vi "Measure, Analyze, and Save I-V of Diodes.vi"() -> ()   [LabVIEW 2020]
doc: "Measure, Analyze, and Save I-V of Diodes.vi contains a state machine that is meant to measure, analyze, and save the I-V characteristics of a diode in series with a resistor on a breadboard using the NI myDAQ data acquisition device. The channel AO0 is used to output a voltage to the breadboard, AI0 is used the measure the voltage across the resistor, and AI1 is used to measure the voltage across the diode. The states are as follows:\n\nInitialize Specifications for Measurement: \nThe user is prompted if they want to input their own measurement specifications or demo the VI with recommended values (for either the linear or log case). The inputted values are checked so that the diode is not put in danger. If the inputted values are safe, the user is sent to the Pre-Measurement state. Otherwise, they are sent to the Input Error state.\n\nPre-Measurement (Calculate Voltage Array):\nThe input values are used to create an array of voltages using the \"Calculate Voltage Array\" sub VI that will be sent to the output of the NI myDAQ device. If the voltage is high enough to exceed the peak current, the creation of the array will cease. Then the user is sent to the Measurement state.\n\nMeasurement:\nThe inputted values are sent the the \"Measure I-V of Diodes\" sub VI. The output voltage, current, and diode voltage measurements are outputted as an array indicator and are plotted to the XY Graph \"I (mA) vs. V_Diode (V)\". A value of 0 V is then dent to the NI myDAQ to turn off the LED after all measurements have been collected. The data is sent to the \"Format Data String\" sub VI which formats the data into a comma-separated values file. The user is prompted on whether they want to choose the filename and path for the saved data or have a default name and path chosen for them. The file path is outputted as an indicator and the user is prompted to either go to the Analysis state or Reset Values and Restart/Stop state.\n\nAnalysis:\nThe current measurements are sent to the \"Indices of Negative Array Elements\" sub VI. The outputted array containing the indices of the negative current values and the voltages are both sent to the \"Remove Elements from Array by Index\" sub VI, which removes any data points with negative current so that they are not out of range for the logarithm of base 10 function. The logarithm of base 10 of the current is then calculated and plotted against the voltage values in the \"Log ( I ( mA ) ) vs. V_Diode ( V )\" XY Graph. A linear best fit is also calculated and plotted. The slope and y-intercept from the best fit line are used to calculate the ideality factor and forward voltage when the current is 1.5 mA. The user is then sent to the Reset Values and Restart/Stop state.\n\nReset Values and Restart/Stop:\nThe user is prompted if they want to restart or stop the state machine. All front panel indicator values are reset.\n\nInput Error:\nThe user is notified that there was an error with their input. Then the state machine restarts."
uses:
  VI State Enum Type Def.ctl
  <vilib>/DAQmx/write.llb/DAQmx Write (Analog DBL 1Chan 1Samp).vi
  <vilib>/DAQmx/create/channels.llb/DAQmx Create Channel (AO-Voltage-Basic).vi
  <vilib>/DAQmx/create/channels.llb/DAQmx Create Channel (AI-Voltage-Basic).vi
  <vilib>/DAQmx/miscellaneous.llb/DAQmx Fill In Error Info.vi
  <vilib>/Analysis/NI_AALPro.lvlib
panel:
  out "Filename Out":path
  out "Room Temperature (K)":dbl
  out "Boltzmann Constant (J/K)":dbl
  out "Electron Charge (C)":dbl
  out "Saturation Current (mA)":dbl
  out "Ideality Factor":dbl
  out "V_F @ 1.5 mA (V)":dbl
  out "Coefficient of Determination":dbl
  out "Y-Intercept":dbl
  out "Slope":dbl
  out "Log ( I (mA) ) vs. V_Diode (V)":cluster{"Y":dbl[], "Y":dbl[]}[](graph)
  out "I (mA) vs. V_Diode (V)":cluster{"Y":dbl[], "Y":dbl[]}[](graph)
  out "I/O Array":dbl[][](array[numeric])
  in  "Stop Measurement":bool
  out "Measurement Specifications":T1
  in  "Stop VI":bool
  # "Measure I-V of Diodes"
  # "V_Applied (V)"
  # "I (mA)"
  # "V_Diode (V)"
  # "Analyze I-V of Diodes"
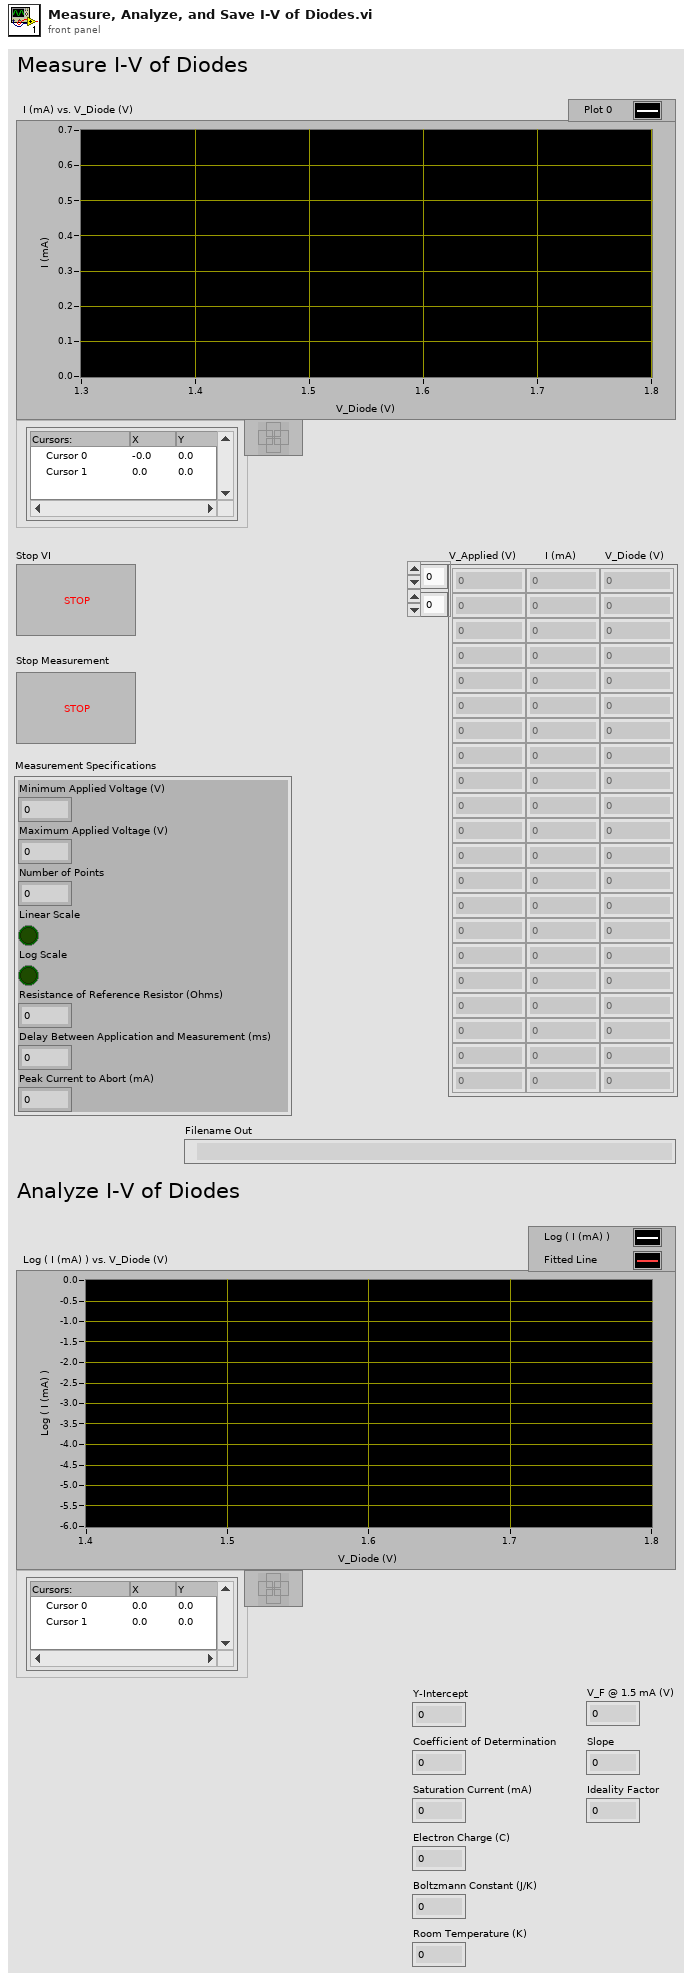
[diagram p1: front panel]
types:
  T1 = cluster{"Minimum Applied Voltage (V)":dbl, "Maximum Applied Voltage (V)":dbl, "Number of Points":i32, "Linear Scale":bool, "Log Scale":bool, "Resistance of Reference Resistor (Ohms)":dbl, "Delay Between Application and Measurement (ms)":dbl, "Peak Current to Abort (mA)":dbl}
  T2 = cluster{"Minimum Applied Voltage (V) (-10 V <= V_min <= 0 V)":dbl, "Maximum Applied Voltage (V) (0 V < V_max <= 10 V)":dbl, "Number of Points to Measure (Integer)":dbl, "Linear Scale":bool, "Log Scale":bool, "Resistance of the Reference Resistor (Ohms)":dbl, "Delay Between Application and Measurement (ms)":dbl, "Peak Current to Abort (mA)":dbl}
  T3 = typedef "VI State Enum Type Def.ctl" = enum16{"Initialize Specifications for Measurement", "Pre-Measurement (Calculate Voltage Array)", "Measurement", "Analysis", "Reset Values and Restart/Stop", "Input Error"}
  T4 = enum16{"open", "replace", "create", "open or create", "replace or create", "replace or create with confirmation"}
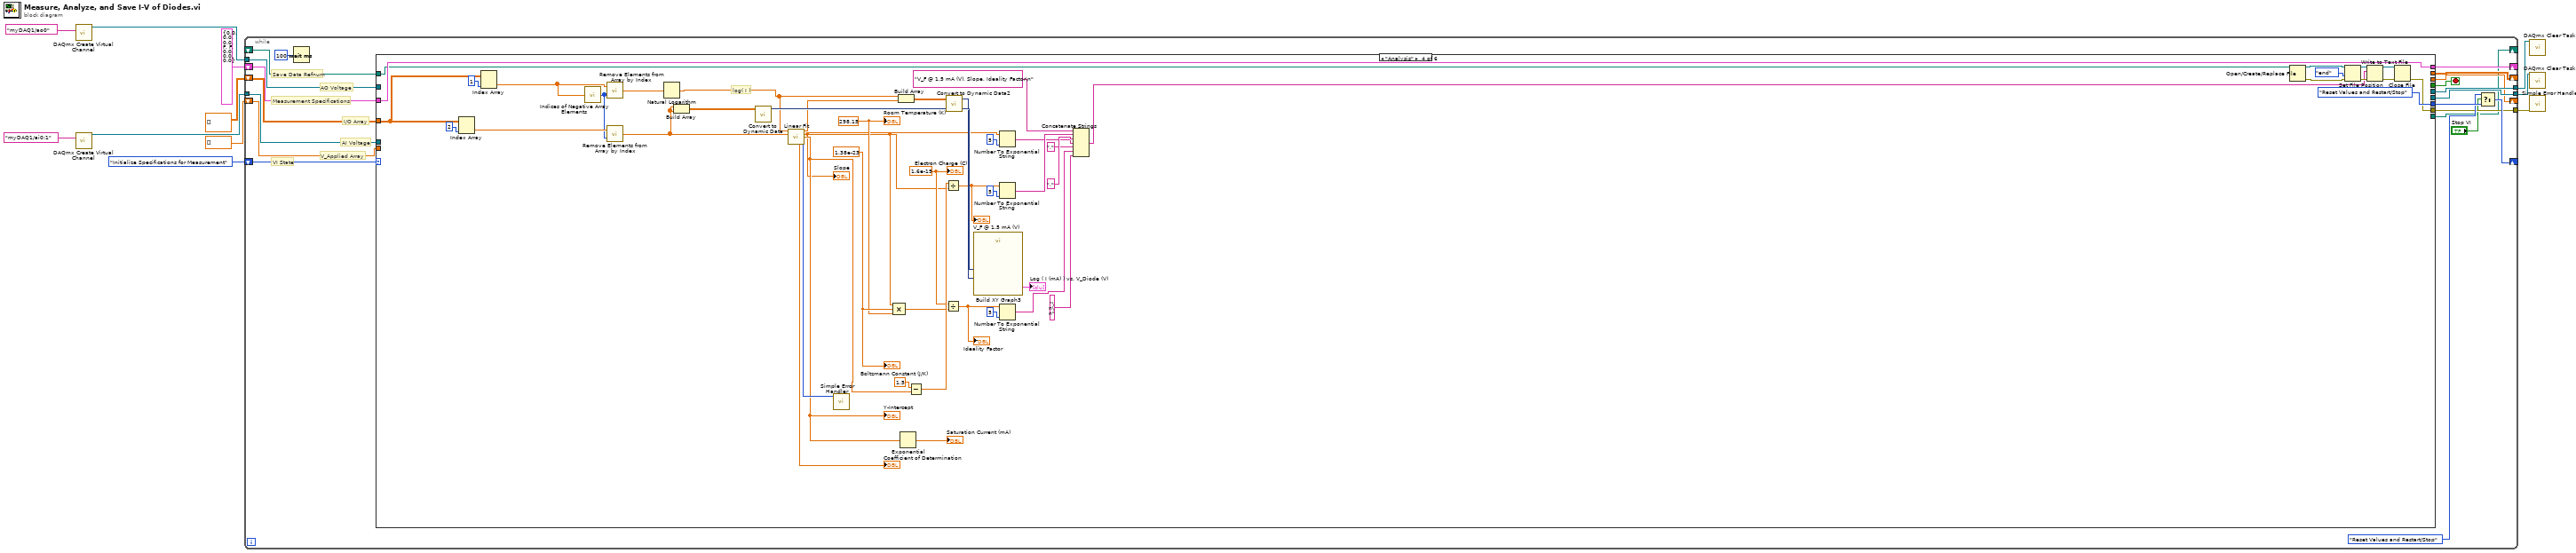
[diagram p0: block diagram]
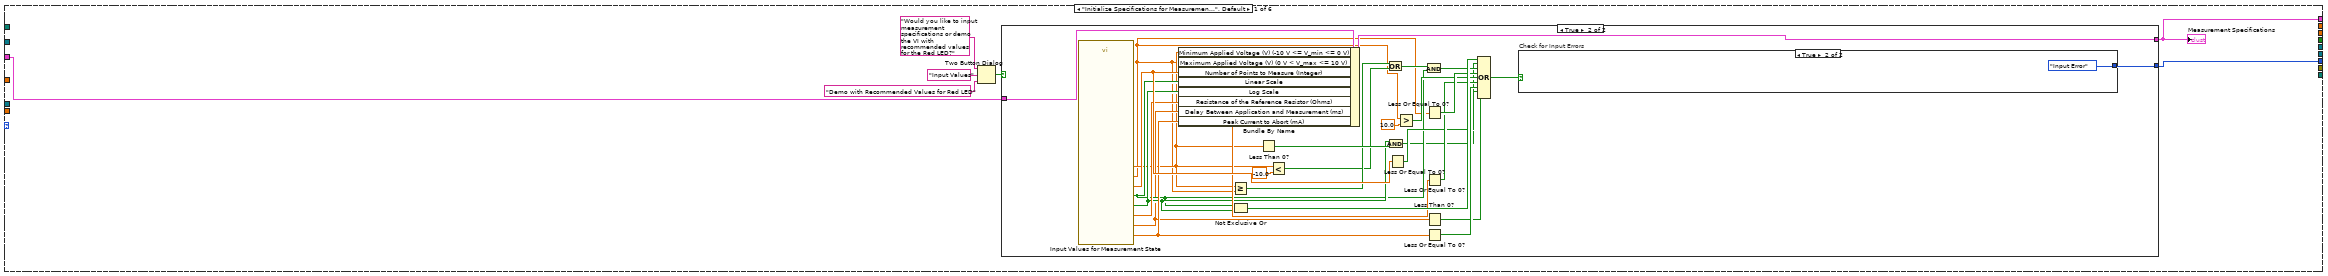
[diagram p2: hidden frame]
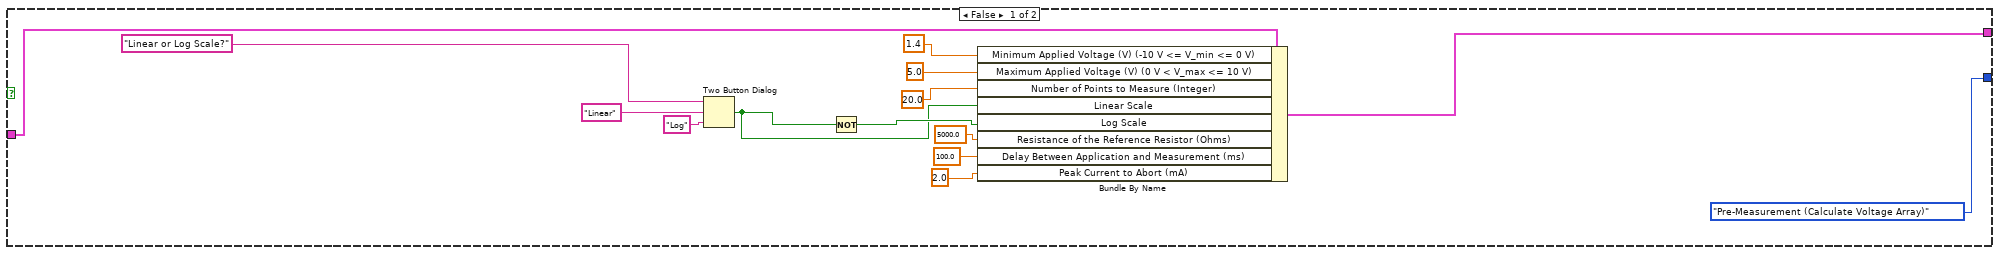
[diagram p3: hidden frame]
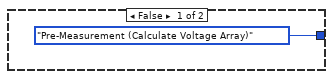
[diagram p4: hidden frame]
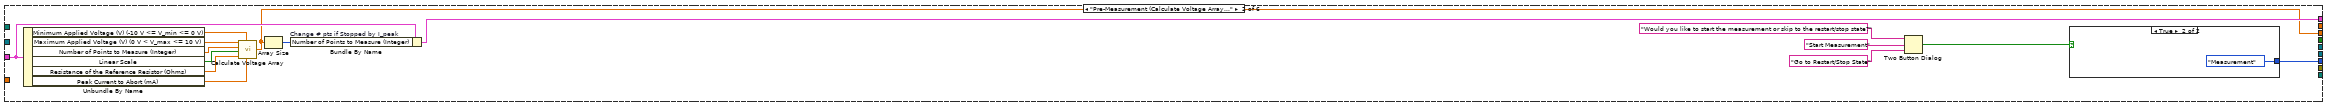
[diagram p5: hidden frame]
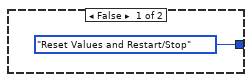
[diagram p6: hidden frame]
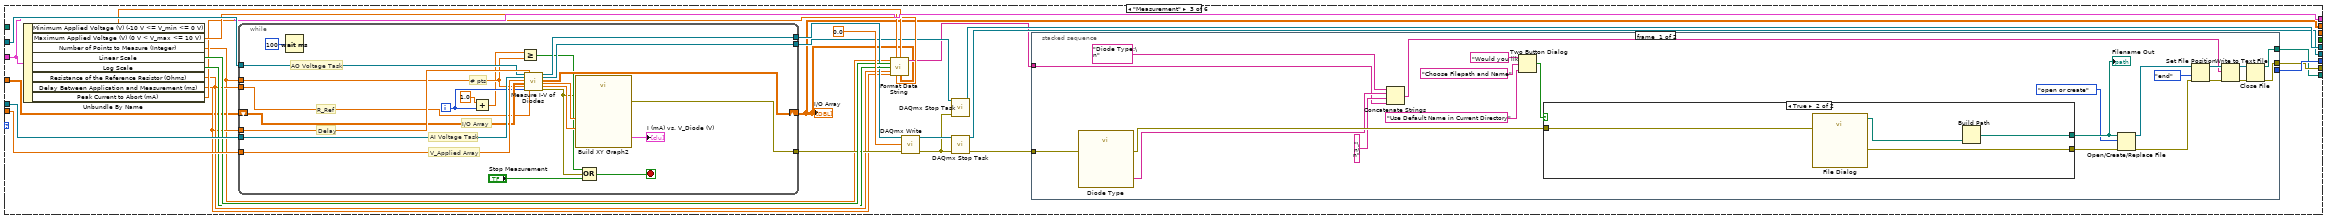
[diagram p7: hidden frame]
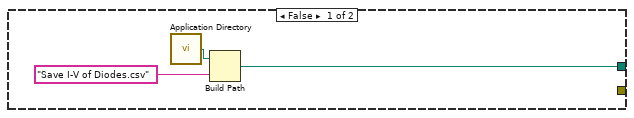
[diagram p8: hidden frame]
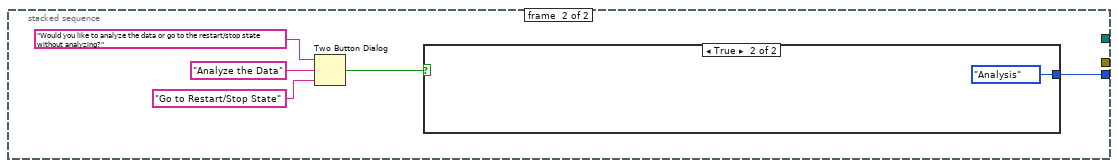
[diagram p9: hidden frame]
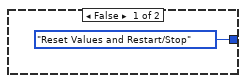
[diagram p10: hidden frame]
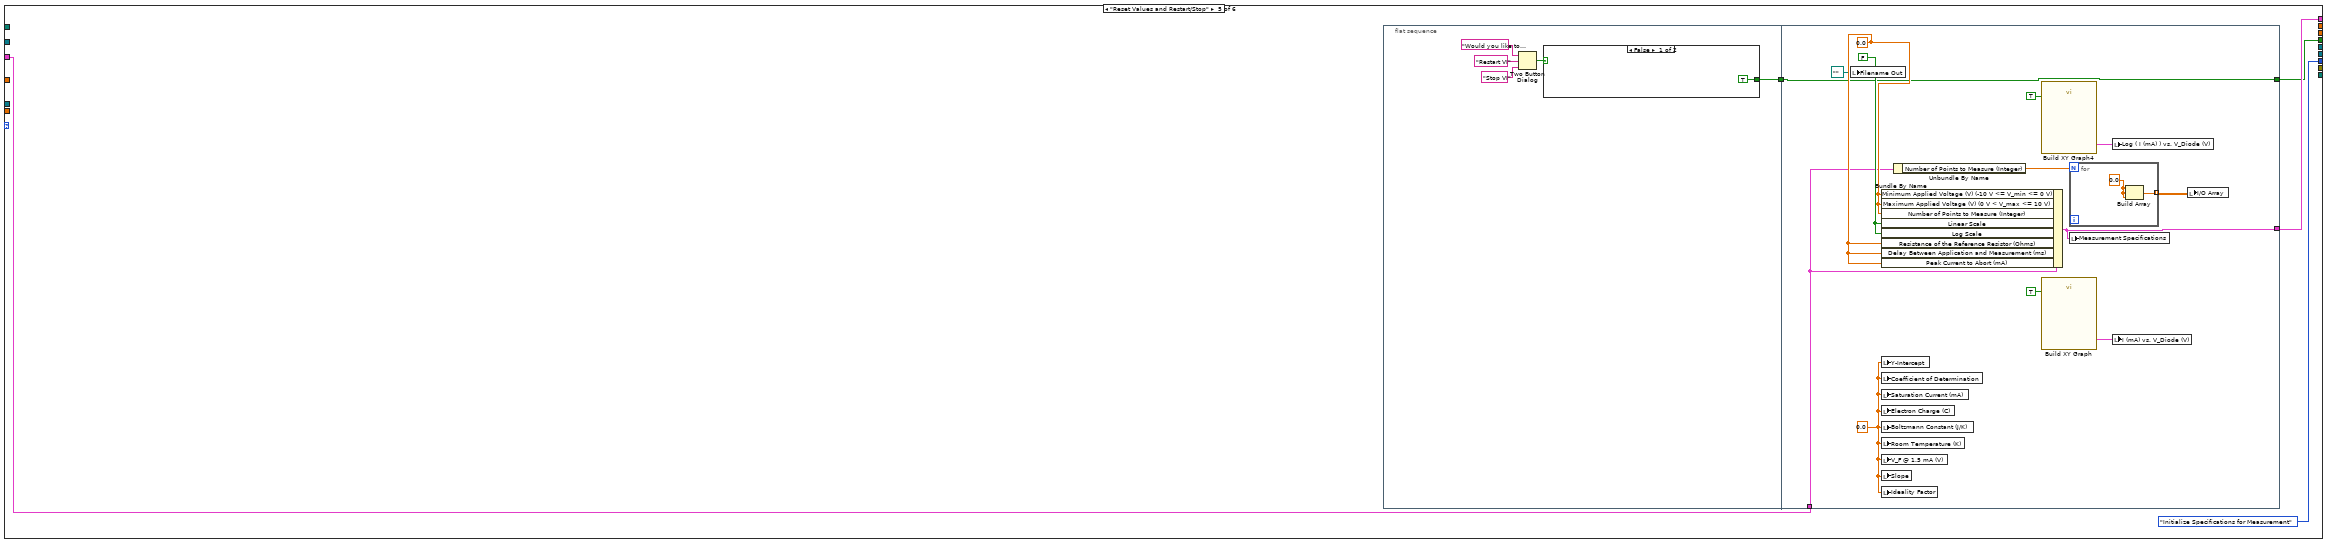
[diagram p11: hidden frame]
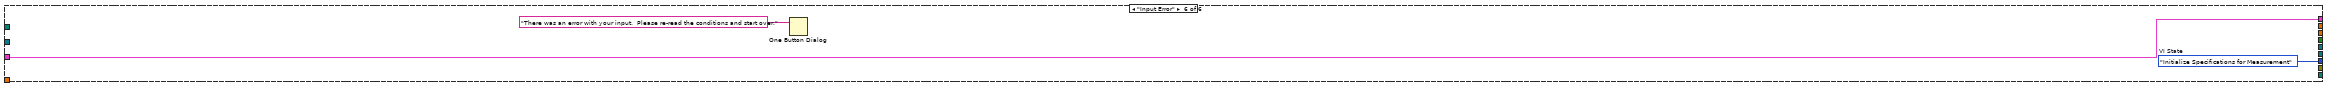
[diagram p13: hidden frame]
diagram:
  n1 = call-poly <vilib>:"DAQmx Create Virtual Channel.vi"("physical channels"=tag "myDAQ1/ao0") -> ("task out"=w5:refnum<k21>)  [unwired: 13 in, 1 out]
  n2 = call-poly <vilib>:"DAQmx Create Virtual Channel.vi"("physical channels"=tag "myDAQ1/ai0:1") -> ("task out"=w8:refnum<k21>)  [unwired: 13 in, 1 out]
  n3 = while {
    shift-right: [w22] -> _
    shift-left: VI_State_Enum_Type_Def."Initialize Specifications for Measurement" ("VI State") -> [w31]
    tunnel: w5 -> [w29]
    tunnel: w8 -> [w28]
    tunnel: [w27] -> w7
    tunnel: [w26] -> w6
    shift-right: [w25] -> _
    shift-left: T2 {"Minimum Applied Voltage (V) (-10 V <= V_min <= 0 V)"=0.0, "Maximum Applied Voltage (V) (0 V < V_max <= 10 V)"=0.0, "Number of Points to Measure (Integer)"=0.0, "Linear Scale"=FALSE, "Log Scale"=FALSE, "Resistance of the Reference Resistor (Ohms)"=0.0, "Delay Between Application and Measurement (ms)"=0.0, "Peak Current to Abort (mA)"=0.0} -> [w24]
    shift-right: [w20] -> _
    shift-left: dbl[] [] ("Voltage Array") -> [w19]
    tunnel: [w18] -> w2
    shift-right: [w17] -> _
    shift-left: dbl[][] [] ("I/O Array Out") -> [w16]
    shift-right: [w13] -> _
    shift-left: _ -> [w12]
    stop <- w15 stop-if-true
    # "Save Data Refnum"
    # "I/O Array"
    # "V_Applied Array"
    # "Measurement Specifications"
    # "AI Voltage"
    # "AO Voltage"
    # "VI State"
    n4 = Wait (ms)(milliseconds to wait=u32 100) -> ()  [unwired: 1 out]
    n5 = case shown="\"Analysis\"" w31 {
      tunnel: [w38 w96 w108 VI_State_Enum_Type_Def."Reset Values and Restart/Stop" ("Measurement State") VI_State_Enum_Type_Def."Initialize Specifications for Measurement" ("VI State") w262] -> w23
      tunnel: w29 -> [_ _ w123 _ _ _]
      tunnel: w28 -> [_ _ w122 _ _ _]
      tunnel: [_ _ w125 _ _ _] -> w27
      tunnel: [_ _ w124 _ _ _] -> w26
      tunnel: [w36 w93 w118 w233 w239 w261] -> w25
      tunnel: w24 -> [w37 w95 w118 w233 w238 w261]
      tunnel: [_ w86 _ _ _ _] -> w20
      tunnel: w19 -> [_ _ w119 _ _ _]
      tunnel: [_ _ w106 w185 _ _] -> w18
      tunnel: [_ _ w101 _ _ _] -> w17
      tunnel: w16 -> [_ _ w100 w231 _ _]
      tunnel: [_ _ _ _ w235 _] -> w15
      tunnel: [_ _ w99 _ _ _] -> w13
      tunnel: w12 -> [_ _ _ w207 _ _]
      frame "Initialize Specifications for Measurement", Default {
        n6 = Two Button Dialog(message="Would you like to input measurement specifications or demo the VI with recommended values for the Red LED?", 1:"Demo with Recommended Values for Red LED" ("F button name (\"Cancel\")"), 2:"Input Values" ("T button name (\"OK\")")) -> (T button?=w32:bool)
        n7 = case shown="True" w32 {
          tunnel: [VI_State_Enum_Type_Def."Pre-Measurement (Calculate Voltage Array)" ("VI State") w79] -> w38
          tunnel: w37 -> [w52 w70]
          tunnel: [w46 w66] -> w36
          frame False {
            n8 = Two Button Dialog(message="Linear or Log Scale?", 1:"Log" ("F button name (\"Cancel\")"), 2:"Linear" ("T button name (\"OK\")")) -> (T button?=w40:bool)
            n9 = Not(x=w40) -> (.not. x?=w41:bool)
            n10 = Bundle By Name(cluster=w52, "Minimum Applied Voltage (V) (-10 V <= V_min <= 0 V)"=1.4, "Maximum Applied Voltage (V) (0 V < V_max <= 10 V)"=5.0, "Number of Points to Measure (Integer)"=20.0, "Linear Scale"=w40, "Log Scale"=w41, "Resistance of the Reference Resistor (Ohms)"=5000.0, "Delay Between Application and Measurement (ms)"=100.0, "Peak Current to Abort (mA)"=2.0) -> (w46:T2)
          }
          frame True {
            n11 = call "Input Values for Measurement State"() -> ("Peak Current to Abort (mA) (I_peak > 0 mA)"=w67:dbl, "Delay Between Application and Measurement (ms) (Delay >= 0 ms)"=w56:dbl, "Resistance of the Reference Resistor (Ohms) (R_ref > 0 Ohms)"=w68:dbl, "Log Scale"=w64:bool, "Linear Scale"=w59:bool, "Number of Points to Measure (Integer) (# pts > 0)"=w69:dbl, "Maximum Applied Voltage (V) (0 V < V_max <= 10 V)"=w53:dbl, "Minimum Applied Voltage (V) (See Above for Conditions)"=w54:dbl)  [unwired: 10 in, 2 out]
            n12 = Bundle By Name(cluster=w70, "Minimum Applied Voltage (V) (-10 V <= V_min <= 0 V)"=w54, "Maximum Applied Voltage (V) (0 V < V_max <= 10 V)"=w53, "Number of Points to Measure (Integer)"=w69, "Linear Scale"=w59, "Log Scale"=w64, "Resistance of the Reference Resistor (Ohms)"=w68, "Delay Between Application and Measurement (ms)"=w56, "Peak Current to Abort (mA)"=w67) -> (w66:T2)
            n13 = Greater Or Equal?(x=w54, y=w53) -> (x >= y?=w63:bool)
            n14 = Not Exclusive Or(1:w64, 2:w59) -> (0:w78:bool)
            n15 = Less Than 0?(x=w54) -> (x < 0?=w65:bool)
            n16 = Less?(x=w54, y=-10.0) -> (x < y?=w62:bool)
            n17 = Or(x=w63, y=w62) -> (x .or. y?=w60:bool)
            n18 = And(x=w64, y=w65) -> (x .and. y?=w55:bool)
            n19 = Less Or Equal To 0?(x=w69) -> (x <= 0?=w71:bool)
            n20 = Greater?(x=w53, y=10.0) -> (0:w74:bool)
            n21 = And(x=w60, y=w59) -> (x .and. y?=w58:bool)
            n22 = Less Or Equal To 0?(x=w53) -> (x <= 0?=w76:bool)
            n23 = Less Or Equal To 0?(x=w68) -> (x <= 0?=w73:bool)
            n24 = Less Than 0?(x=w56) -> (x < 0?=w57:bool)
            n25 = Less Or Equal To 0?(x=w67) -> (x <= 0?=w72:bool)
            n26 = Compound Arithmetic op=OR(w78, w55, w58, w76, w74, w73, w72, w71, w57) -> (w77:bool)
            n27 = case "Check for Input Errors" shown="True" w77 {
              tunnel: [VI_State_Enum_Type_Def."Pre-Measurement (Calculate Voltage Array)" ("Measurement State") VI_State_Enum_Type_Def."Input Error" ("Measurement State")] -> w79
              frame False {
              }
              frame True {
              }
            }
          }
        }
        "Measurement Specifications" <- w36
      }
      frame "Pre-Measurement (Calculate Voltage Array)" {
        n28 = Unbundle By Name(w95) -> ("Minimum Applied Voltage (V) (-10 V <= V_min <= 0 V)"=w92:dbl, "Maximum Applied Voltage (V) (0 V < V_max <= 10 V)"=w91:dbl, "Number of Points to Measure (Integer)"=w90:dbl, "Linear Scale"=w89:bool, "Resistance of the Reference Resistor (Ohms)"=w88:dbl, "Peak Current to Abort (mA)"=w87:dbl)
        n29 = call "Calculate Voltage Array.vi"("I_peak"=w87, "V_min"=w92, "R_ref"=w88, "Scale (True == Linear, False == Log)"=w89, "# pts"=w90, "V_max"=w91) -> ("Voltage Array"=w86:dbl[])
        n30 = Array Size(array=w86) -> (size(s)=w94:i32)
        n31 = Bundle By Name "Change # pts if Stopped by I_peak"(cluster=w95, "Number of Points to Measure (Integer)"=w94) -> (w93:T2)
        n32 = Two Button Dialog(message="Would you like to start the measurement or skip to the restart/stop state?", 1:"Go to Restart/Stop State" ("F button name (\"Cancel\")"), 2:"Start Measurement" ("T button name (\"OK\")")) -> (T button?=w85:bool)
        n33 = case shown="True" w85 {
          tunnel: [VI_State_Enum_Type_Def."Reset Values and Restart/Stop" ("Measurement State") VI_State_Enum_Type_Def."Measurement" ("Measurement State")] -> w96
          frame False {
          }
          frame True {
          }
        }
      }
      frame "Measurement" {
        n34 = Unbundle By Name(w118) -> ("Minimum Applied Voltage (V) (-10 V <= V_min <= 0 V)"=w117:dbl, "Maximum Applied Voltage (V) (0 V < V_max <= 10 V)"=w116:dbl, "Number of Points to Measure (Integer)"=w103:dbl, "Linear Scale"=w115:bool, "Log Scale"=w114:bool, "Resistance of the Reference Resistor (Ohms)"=w105:dbl, "Delay Between Application and Measurement (ms)"=w104:dbl, "Peak Current to Abort (mA)"=w113:dbl)
        n35 = while {
          tunnel: w104 -> [w182]
          tunnel: w123 -> [w181]
          tunnel: w122 -> [w180]
          tunnel: w119 -> [w179]
          tunnel: w103 -> [w171]
          shift-right: [w174] -> w101
          shift-left: w100 -> [w178]
          tunnel: w105 -> [w177]
          tunnel: [w176] -> w111
          tunnel: [w175] -> w110
          tunnel: [w163] -> w109
          i -> [w166]
          stop <- w169 stop-if-true
          # "R_Ref"
          # "I/O Array"
          # "V_Applied Array"
          # "# pts"
          # "AI Voltage Task"
          # "AO Voltage Task"
          # "Delay"
          n36 = Wait (ms)(milliseconds to wait=u32 100) -> ()  [unwired: 1 out]
          n37 = Add(x=1.0, y=w166) -> (x+y=w165:dbl)
          n38 = Greater Or Equal?(x=w165, y=w171) -> (x >= y?=w168:bool)
          n39 = call "Measure I-V of Diodes.vi"("AO Task In"=w181, "AI Task In"=w180, "V_App Array"=w179, "I/O Array In"=w178, "# pts"=w171, "index"=w166, "Delay"=w182, "R_Ref"=w177) -> ("AO Task Out"=w176:refnum<k21>, "AI Task Out"=w175:refnum<k21>, "I/O Array Out"=w174:dbl[][], "X Input"=w173:dbl, "Y Input"=w172:dbl, "error out"=w164:errorcluster)  [unwired: 6 in]
          n40 = call "Build XY Graph2"("error in (no error)"=w164, "Y Input"=w172, "X Input"=w173) -> ("error out"=w163:errorcluster, "XY Graph"=→"I (mA) vs. V_Diode (V)":cluster{"X":dbl[], "Y":dbl[]}[])  [unwired: 7 in]
          n41 = Compound Arithmetic op=OR(w168, w164, "Stop Measurement") -> (w169:bool)
        }
        "I/O Array" <- w101
        n42 = call "Format Data String.vi"("# pts"=w103, "V_max"=w116, "V_min"=w117, "Linear Scale"=w115, "Log Scale"=w114, "R_Ref"=w105, "Delay"=w104, "I_Peak"=w113, "I/O Array"=w101) -> ("Formatted Data String"=w107:string)  [unwired: 6 in]
        n43 = call-poly <vilib>:"DAQmx Write.vi"("task/channels in"=w111, "data"=0.0, "error in"=w109) -> ("task out"=w121:refnum<k21>, "error out"=w112:errorcluster)  [unwired: 10 in, 1 out]
        n44 = call <vilib>:"DAQmx Stop Task.vi"("task/channels in"=w110, "error in"=w112) -> ("task out"=w125:refnum<k21>)  [unwired: 12 in, 1 out]
        n45 = call <vilib>:"DAQmx Stop Task.vi"("task/channels in"=w121, "error in"=w112) -> ("task out"=w124:refnum<k21>, "error out"=w102:errorcluster)  [unwired: 12 in]
        n46 = stacked-sequence {
          tunnel: [_ w160] -> w108
          tunnel: [w134 _] -> w106
          tunnel: w107 -> [w127 _]
          tunnel: w102 -> [w132 _]
          tunnel: [w133 _] -> w99
          frame #0 {
            n47 = call "Diode Type"("error in (no error)"=w132) -> ("Diode Type:"=w129:string, "error out"=w131:errorcluster)  [unwired: 16 in, 1 out]
            n48 = Concatenate Strings("Diode Type:\n" ("string"), w129, "\n\n" ("string"), w127) -> (w126:string)
            n49 = Two Button Dialog(message="Would you like to choose the name and file path of the saved data or would you like to save it under a default name in the current directory?", 1:"Use Default Name in Current Directory" ("F button name (\"Cancel\")"), 2:"Choose Filepath and Name" ("T button name (\"OK\")")) -> (T button?=w141:bool)
            n50 = case shown="True" w141 {
              tunnel: [w150 w155] -> w147
              tunnel: [_ w153] -> w135
              tunnel: w131 -> [_ w152]
              frame False {
                n51 = call <vilib>:"Application Directory.vi"() -> ("Application Directory"=w149:path)
                n52 = Build Path(base path=w149, name or relative path="Save I-V of Diodes.csv") -> (appended path=w150:path)
              }
              frame True {
                n53 = call "File Dialog"("error in"=w152) -> ("selected path"=w154:path, "error out"=w153:errorcluster)  [unwired: 11 in, 2 out]
                n54 = Build Path(name or relative path=w154) -> (appended path=w155:path)  [unwired: 1 in]
              }
            }
            "Filename Out" <- w147
            n55 = Open/Create/Replace File(file path (use dialog)=w147, error in=w135, operation (0:open)=T4."open or create") -> (refnum out=w144:refnum<file>, error out=w148:errorcluster)  [unwired: 3 in, 1 out]
            n56 = Set File Position(refnum=w144, from (0:start)=enum16{"start", "end", "current"}."end", error in=w148) -> (refnum out=w145:refnum<file>, error out=w146:errorcluster)  [unwired: 1 in]
            n57 = Write to Text File(file (use dialog)=w145, text=w126, error in=w146) -> (refnum out=w143:refnum<file>, error out=w142:errorcluster)  [unwired: 1 in, 1 out]
            n58 = Close File(refnum=w143, error in=w142) -> (path=w133:path, error out=w134:errorcluster)
          }
          frame #1 {
            n59 = Two Button Dialog(message="Would you like to analyze the data or go to the restart/stop state without analyzing?", 1:"Go to Restart/Stop State" ("F button name (\"Cancel\")"), 2:"Analyze the Data" ("T button name (\"OK\")")) -> (T button?=w156:bool)
            n60 = case shown="True" w156 {
              tunnel: [VI_State_Enum_Type_Def."Reset Values and Restart/Stop" ("Measurement State") VI_State_Enum_Type_Def."Analysis" ("Measurement State")] -> w160
              frame False {
              }
              frame True {
              }
            }
          }
        }
      }
      frame "Analysis" {
        w215 = 298.15 ("Room Temperature (K)")
        w216 = 1.38e-23 ("Boltzmann Constant (J/K)")
        w217 = 1.6e-19 ("Electron Charge (C)")
        # "log( I )"
        n61 = Index Array(array=w231, index (col)=2 ("disabled index (col)")) -> (element=w211:dbl[])  [unwired: 1 in]
        n62 = Index Array(array=w231, index (col)=1 ("disabled index (col)")) -> (element=w213:dbl[])  [unwired: 1 in]
        n63 = call "Indices of Negative Array Elements.vi"("Array In"=w213) -> ("Indices"=w210:i32[])
        n64 = call "Remove Elements from Array by Index.vi"("Indices"=w210, "Array In"=w213) -> ("Array Out 2"=w212:dbl[])
        n65 = call "Remove Elements from Array by Index.vi"("Indices"=w210, "Array In"=w211) -> ("Array Out 2"=w208:dbl[])
        n66 = Natural Logarithm(1:w212) -> (0:w225:dbl[])
        n67 = Build Array(w208, w208) -> (w209:dbl[][])
        n68 = call "Convert to Dynamic Data"("2D Array"=w209) -> ("Dynamic Data Type"=w226:dynamicdata)  [unwired: 3 in]
        n69 = call <vilib>:"Linear Fit.vi"("Y"=w225, "X"=w208) -> ("Best Linear Fit"=w224:dbl[], "slope"=w193:dbl, "intercept"=w219:dbl, "residue"=→"Coefficient of Determination":dbl, "error"=w227:i32)  [unwired: 9 in]
        "Slope" <- w193
        "Y-Intercept" <- w219
        n70 = call <vilib>:"Simple Error Handler.vi"("error code (no error:0)"=w227) -> ()  [unwired: 4 in, 5 out]
        n71 = Compound Arithmetic op=MULTIPLY(w193, w216, w215) -> (w214:dbl)
        n72 = Build Array(w225, w224) -> (w223:dbl[][])
        n73 = Exponential(1:w219) -> (0:→"Saturation Current (mA)":dbl)
        n74 = Subtract(x=1.5, y=w219) -> (x-y=w220:dbl)
        n75 = Divide(x=w220, y=w193) -> (x/y=w197:dbl)
        "V_F @ 1.5 mA (V)" <- w197
        n76 = Divide(x=w217, y=w214) -> (x/y=w189:dbl)
        "Ideality Factor" <- w189
        n77 = call "Convert to Dynamic Data2"("2D Array"=w223) -> ("Dynamic Data Type"=w222:dynamicdata)  [unwired: 3 in]
        n78 = call "Build XY Graph3"("Y Input"=w222, "X Input"=w226) -> ("XY Graph"=→"Log ( I (mA) ) vs. V_Diode (V)":cluster{"X":dbl[], "Y":dbl[]}[])  [unwired: 8 in, 1 out]
        n79 = Number To Exponential String(number=w193, precision (6)=i16 5) -> (E-format string=w192:string)  [unwired: 2 in]
        n80 = Number To Exponential String(number=w197, precision (6)=i16 5) -> (E-format string=w196:string)  [unwired: 2 in]
        n81 = Number To Exponential String(number=w189, precision (6)=i16 5) -> (E-format string=w188:string)  [unwired: 2 in]
        n82 = Concatenate Strings("V_F @ 1.5 mA (V), Slope, Ideality Factor\n" ("string"), w196, "," ("string"), w192, "," ("string"), w188, "\n\n" ("string")) -> (w186:string)
        n83 = Open/Create/Replace File(file path (use dialog)=w207) -> (refnum out=w202:refnum<file>, error out=w201:errorcluster)  [unwired: 5 in, 1 out]
        n84 = Set File Position(refnum=w202, from (0:start)=enum16{"start", "end", "current"}."end", error in=w201) -> (refnum out=w200:refnum<file>, error out=w199:errorcluster)  [unwired: 1 in]
        n85 = Write to Text File(file (use dialog)=w200, text=w186, error in=w199) -> (refnum out=w205:refnum<file>, error out=w206:errorcluster)  [unwired: 1 in, 1 out]
        n86 = Close File(refnum=w205, error in=w206) -> (error out=w185:errorcluster)  [unwired: 1 out]
        "Electron Charge (C)" <- w217
        "Boltzmann Constant (J/K)" <- w216
        "Room Temperature (K)" <- w215
      }
      frame "Reset Values and Restart/Stop" {
        n87 = flat-sequence {
          tunnel: [w240] -> w236
          tunnel: [w256] -> w239
          tunnel: w238 -> [w255]
          tunnel: w236 -> [w247]
          tunnel: [w247] -> w235
          frame #0 {
            n88 = Two Button Dialog(message="Would you like to reset the values and restart the VI or stop the VI?", 1:"Stop VI" ("F button name (\"Cancel\")"), 2:"Restart VI" ("T button name (\"OK\")")) -> (T button?=w244:bool)
            n89 = case shown="False" w244 {
              tunnel: [TRUE _] -> w240
              frame False {
              }
              frame True {
              }
            }
          }
          frame #1 {
            w248 = 0.0 ("Y-Intercept")
            w257 = 0.0 ("Minimum Applied Voltage (V) (-10 V <= V_min <= 0 V)")
            w258 = FALSE ("Linear Scale")
            n90 = local write "Filename Out"(path "" ("Filename Out")) -> ()
            n91 = Bundle By Name(cluster=w255, "Minimum Applied Voltage (V) (-10 V <= V_min <= 0 V)"=w257, "Maximum Applied Voltage (V) (0 V < V_max <= 10 V)"=w257, "Number of Points to Measure (Integer)"=w257, "Linear Scale"=w258, "Log Scale"=w258, "Resistance of the Reference Resistor (Ohms)"=w257, "Delay Between Application and Measurement (ms)"=w257, "Peak Current to Abort (mA)"=w257) -> (w256:T2)
            n92 = local write "Y-Intercept"(w248) -> ()
            n93 = local write "Coefficient of Determination"(w248) -> ()
            n94 = local write "Saturation Current (mA)"(w248) -> ()
            n95 = local write "Electron Charge (C)"(w248) -> ()
            n96 = local write "Boltzmann Constant (J/K)"(w248) -> ()
            n97 = local write "Room Temperature (K)"(w248) -> ()
            n98 = local write "V_F @ 1.5 mA (V)"(w248) -> ()
            n99 = local write "Slope"(w248) -> ()
            n100 = local write "Ideality Factor"(w248) -> ()
            n101 = Unbundle By Name(w255) -> ("Number of Points to Measure (Integer)"=w254:dbl)
            n102 = call "Build XY Graph4"("Reset"=TRUE) -> ("XY Graph"=w249:cluster{"X":dbl[], "Y":dbl[]}[])  [unwired: 9 in, 1 out]
            n103 = call "Build XY Graph"("Reset"=TRUE) -> ("XY Graph"=w252:cluster{"X":dbl[], "Y":dbl[]}[])  [unwired: 9 in, 1 out]
            n104 = for {
              N: w254 -> [_]
              tunnel: [w259] -> w253 mode=indexing
              w260 = 0.0 ("element")
              n105 = Build Array(w260, w260, w260) -> (w259:dbl[])
            }
            n106 = local write "Measurement Specifications"(w256) -> ()
            n107 = local write "Log ( I (mA) ) vs. V_Diode (V)"(w249) -> ()
            n108 = local write "I (mA) vs. V_Diode (V)"(w252) -> ()
            n109 = local write "I/O Array"(w253) -> ()
          }
        }
      }
      frame "Input Error" {
        w262 = VI_State_Enum_Type_Def."Initialize Specifications for Measurement"  # VI State
        n110 = One Button Dialog(message="There was an error with your input.  Please re-read the conditions and start over.") -> ()  [unwired: 1 in, 1 out]
      }
    }
    n111 = Select(t=VI_State_Enum_Type_Def."Reset Values and Restart/Stop" ("VI State"), s="Stop VI", f=w23) -> (s? t:f=w22:T3)
  }
  n112 = call <vilib>:"DAQmx Clear Task.vi"("task in"=w7) -> ()  [unwired: 14 in, 1 out]
  n113 = call <vilib>:"DAQmx Clear Task.vi"("task in"=w6) -> ()  [unwired: 14 in, 1 out]
  n114 = call <vilib>:"Simple Error Handler.vi"("error in (no error)"=w2) -> ()  [unwired: 4 in, 5 out]
